vi "3D_Traverse_move.vi"(0 "Mode":T4=enum."Read traverse position", 1 "Position":sgl[](array[numeric])=[0.0, 0.0, 0.0] format="%#.2f", 2 "Extra command String":string, 3 "Work in Tunnel Coordinates":T2, 4 "Home":T1, 5 "Simulate/Run":T3=enum."Run VI", 6 "Route Checking?":bool=TRUE, 7 "Traverse name":string, 8 "Display Trav 2 Trav Error":bool=TRUE, 9 "Backlash Compensation?":bool=TRUE, 10 "Row Number":i32=-1, 11 "Last Part of Move?":bool=TRUE, 13 "Currently on Point":i32=-1) -> (12 "Model:    Roll        Pitch         Yaw  (deg)":sgl[](array[numeric]) caption="ModelRollPitchYaw (deg)" format="%#.2f", 14 "Trav Position achieved":sgl[](array[numeric]) format="%#.2f", 19 "Error String":string)   [LabVIEW 2016]
uses:
  Trav_mode.ctl
  Controls/User_Specific_mode.ctl
  Controls/Tunnel_Coordinates.ctl
  Controls/Home.ctl
  ADAM Client/Sub VIs/ADAM Controls/Quick_local_ADAM_Table.ctl
  Route mapping/Route_Display_Mode.ctl
  Controls/In_Range.ctl
  Globals/Trav_pos_global.vi
  Globals/Preference_global.vi
  Globals/Constants_global.vi
  Route mapping/Route_mapping_global.vi
panel:
  in  "Position Offset":sgl[](array[numeric])=[0.0, 0.0, 0.0] step=1 format="%#.2f"
  out "Traverses Available":string[](array[string])
  in  "Traverse":u16(ring) items=["EnFlo_Stack", "EnFlo_Trav1", "EnFlo_Trav3", "EnFlo_Trav4", "EnFlo_Tunnel", "EnFlo_Turntable"]
  # "X                Y                   Z"
  # "X                Y                   Z"
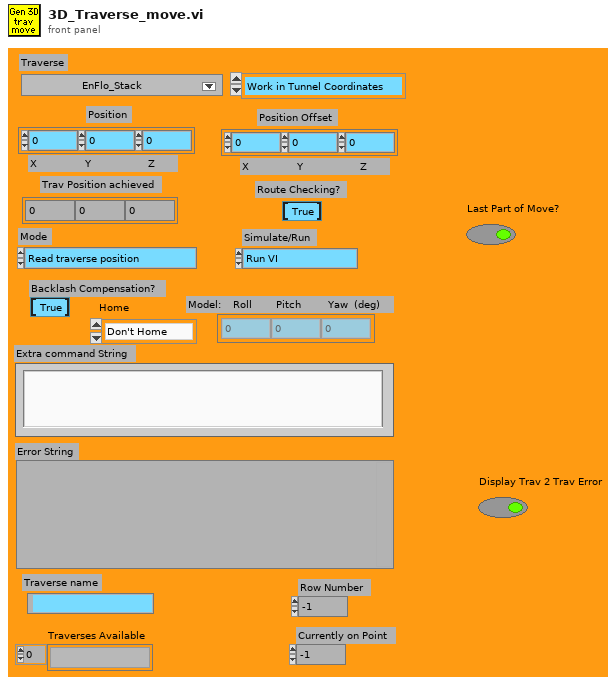
[diagram p1: front panel]
types:
  T1 = typedef "Home.ctl" = enum16{"Don't Home", "Home  +X", "Home  -X", "Home  +Y", "Home  -Y", "Home  +Z", "Home  -Z"}
  T2 = typedef "Tunnel_Coordinates.ctl" = enum16{"Work in Tunnel Coordinates", "Work in Model Coordinates"}
  T3 = typedef "User_Specific_mode.ctl" = enum16{"Check VI only", "Run VI"}
  T4 = typedef "Trav_mode.ctl" = enum16{"Move traverse", "Read traverse position", "Teach Position"}
  T5 = enum16{"To Traverse Coordinates", "To User Coordinates"}
  T6 = typedef "Quick_local_ADAM_Table.ctl" = enum16{"Read Global", "Load Global From ADAM Table", "Write Global"}
  T7 = typedef "Route_Display_Mode.ctl" = enum16{"Display View Always", "Display View on Crash"}
  T8 = typedef "In_Range.ctl" = enum16{"%", "±", "% & ±"}
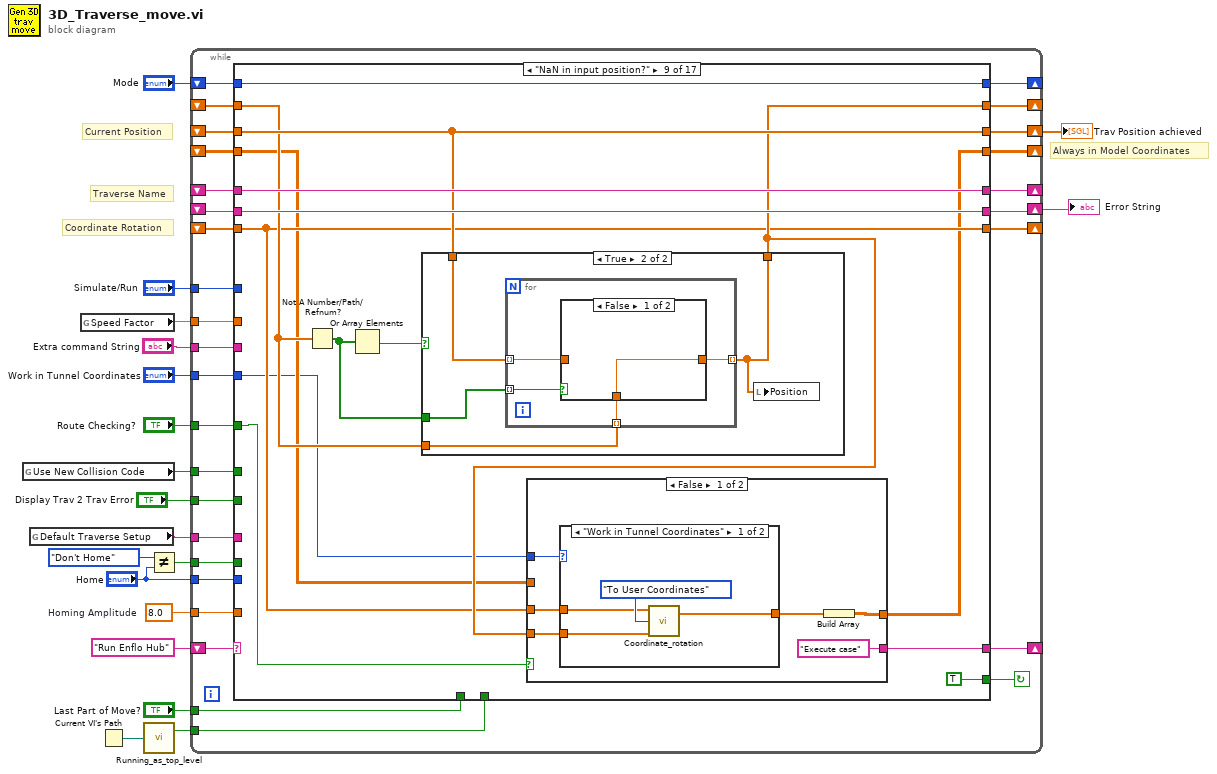
[diagram p0: block diagram]
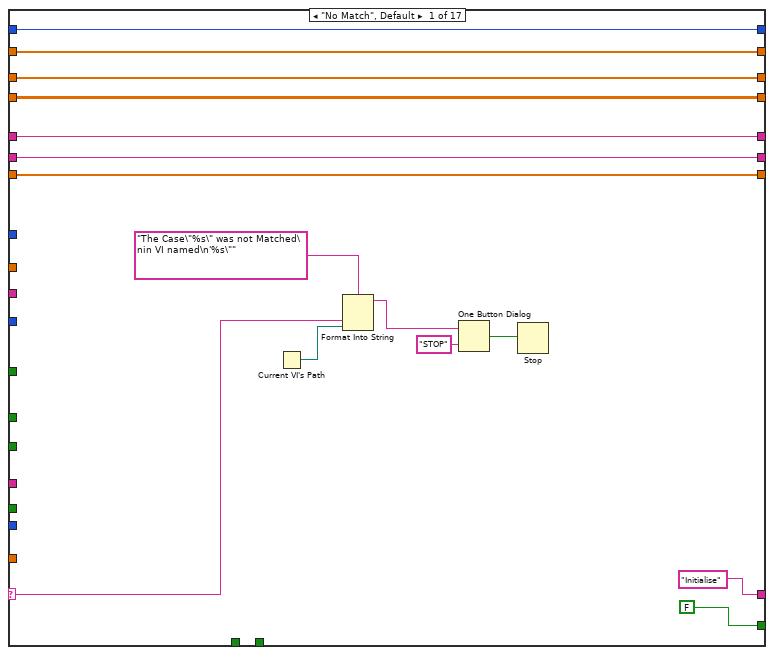
[diagram p2: hidden frame]
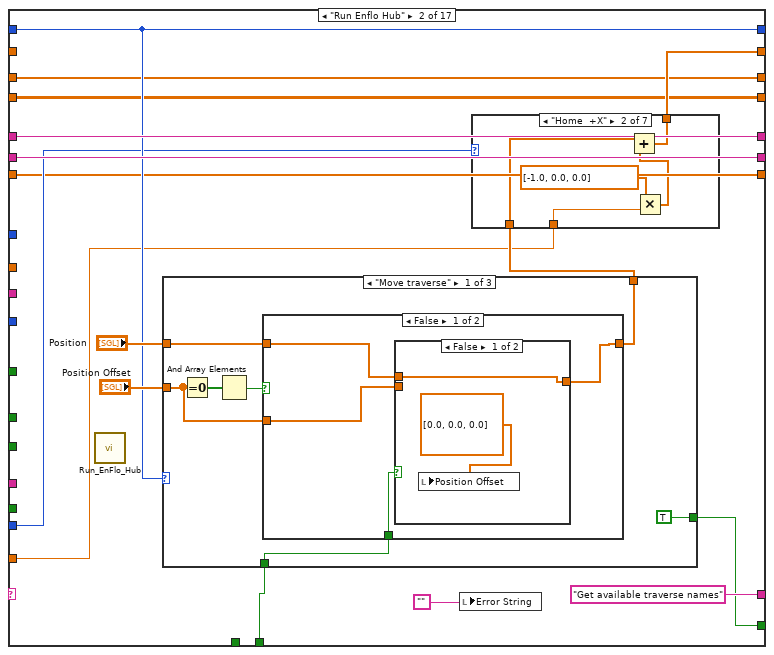
[diagram p3: hidden frame]
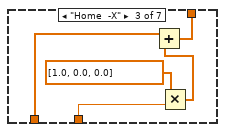
[diagram p5: hidden frame]
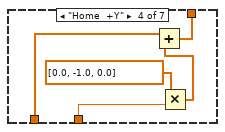
[diagram p6: hidden frame]
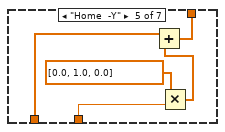
[diagram p7: hidden frame]
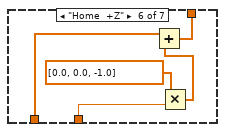
[diagram p8: hidden frame]
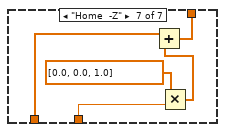
[diagram p9: hidden frame]
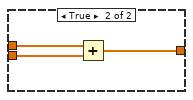
[diagram p10: hidden frame]
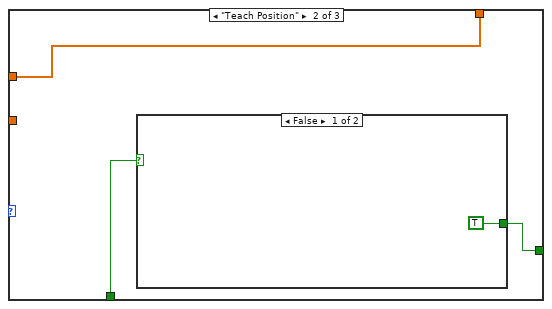
[diagram p12: hidden frame]
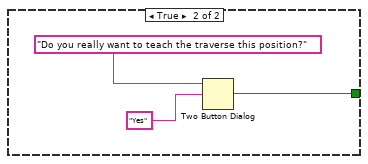
[diagram p13: hidden frame]
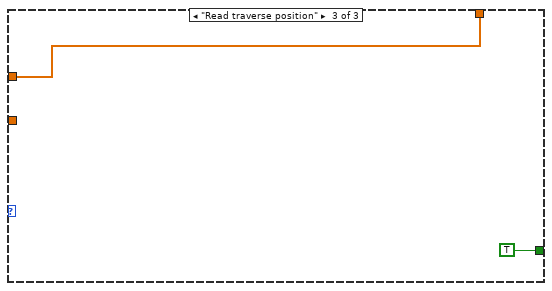
[diagram p14: hidden frame]
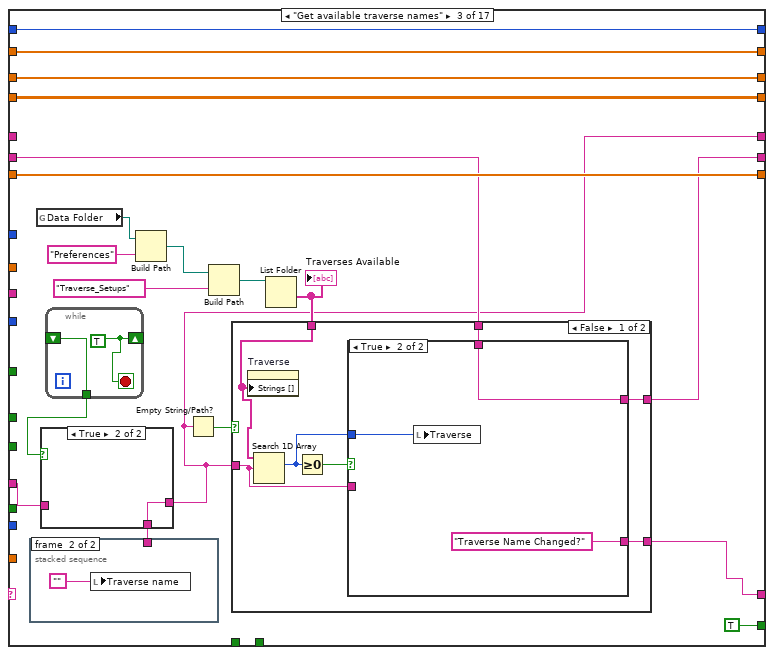
[diagram p15: hidden frame]
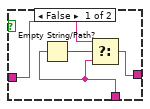
[diagram p16: hidden frame]
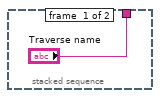
[diagram p17: hidden frame]
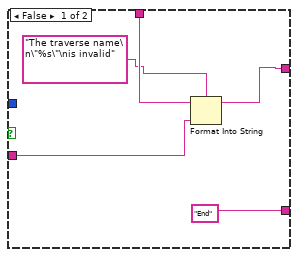
[diagram p18: hidden frame]
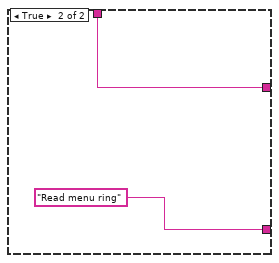
[diagram p19: hidden frame]
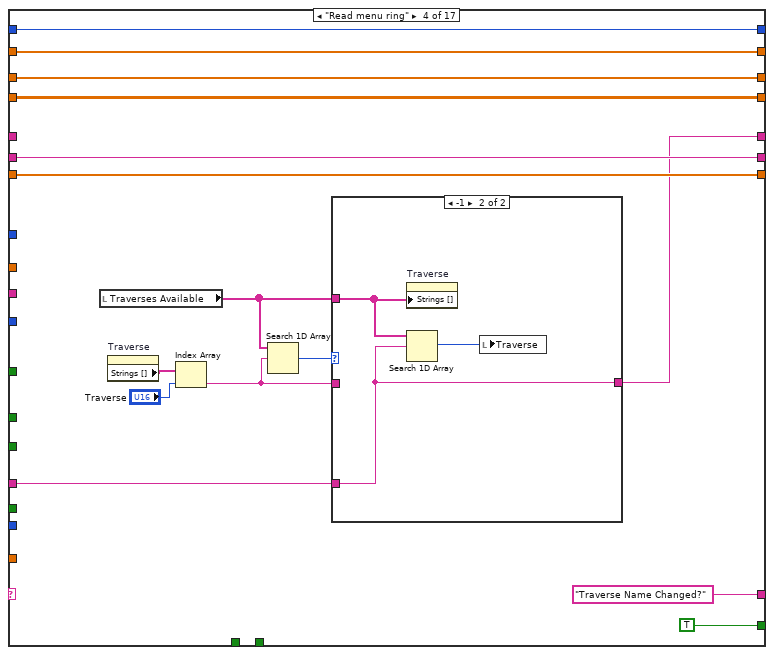
[diagram p20: hidden frame]
diagram:
  w10 = sgl 8.0  # Homing Amplitude
  # "Always in Model Coordinates"
  # "Current Position"
  # "Coordinate Rotation"
  # "Traverse Name"
  n1 = global read "Preference_global.vi" "Use New Collision Code"() -> (w6:bool)
  n2 = global read "Trav_pos_global.vi" "Default Traverse Setup"() -> (w12:string)
  n3 = global read "Trav_pos_global.vi" "Speed Factor"() -> (w16:sgl)
  n4 = Current VI's Path() -> (path=w4:path)
  n5 = call "Running_as_top_level.vi"("Vi path name"=w4) -> ("Top Level"=w3:bool)  [unwired: 1 out]
  n6 = Not Equal?(x=Home."Don't Home" ("Home"), y="Home") -> (x != y?=w7:bool)
  n7 = while {
    shift-left: "Run Enflo Hub" -> [w47]
    shift-right: [w48] -> _
    shift-right: [w45] -> _
    shift-left: _ -> [w43]
    tunnel: "Simulate/Run" -> [w46]
    shift-right: [w44] -> w17
    shift-left: _ -> [w42]
    shift-right: [w40] -> _
    shift-left: _ -> [w41]
    shift-right: [w37] -> _
    shift-left: _ -> [w36]
    shift-right: [w38] -> w13
    shift-left: _ -> [w39]
    tunnel: w16 -> [w35]
    tunnel: "Work in Tunnel Coordinates" -> [w34]
    tunnel: "Route Checking?" -> [w33]
    tunnel: w12 -> [w32]
    shift-right: [w31] -> _
    shift-left: _ -> [w30]
    shift-right: [w28] -> _
    shift-left: "Mode" -> [w29]
    tunnel: "Home" -> [w27]
    tunnel: w10 -> [w26]
    tunnel: w7 -> [w25]
    tunnel: w6 -> [w24]
    tunnel: "Last Part of Move?" -> [w23]
    tunnel: w3 -> [w22]
    tunnel: "Extra command String" -> [w21]
    tunnel: "Display Trav 2 Trav Error" -> [w20]
    stop <- w49 continue-if-true
    n8 = case shown="\"NaN in input position?\"" w47 {
      selector: w47 -> [w50 _ _ _ _ _ _ _ _ _ _ _ _ _ _ _ _]
      tunnel: [FALSE w76 TRUE TRUE TRUE TRUE w292 TRUE ("T button?") TRUE ("T button?") w395 TRUE w550 w577 TRUE TRUE TRUE FALSE] -> w49
      tunnel: ["Initialise" "Get available traverse names" w148 "Traverse Name Changed?" "Mode" w261 w299 "NaN in input position?" w353 w396 w449 "Display Traverse Views" w584 "Update Position Globals" "Tidy up" "End" "End"] -> w48
      tunnel: w46 -> [_ _ _ _ w226 w262 w304 _ _ w404 w445 _ w582 _ w681 w723 w821]
      tunnel: [w57 w79 w140 w184 w221 w254 w308 w340 w366 w406 w444 w555 w589 w631 w680 w728 w817] -> w45
      tunnel: [w56 w78 w146 w196 "" w263 w293 "" w363 w399 w453 w547 w586 w616 w684 w730 w824] -> w44
      tunnel: w43 -> [w57 w79 _ _ w221 w254 w308 w340 w366 w406 w444 w555 w589 w631 w680 w728 w817]
      tunnel: w42 -> [w56 w78 w145 w196 _ w263 _ _ w363 w401 _ w548 w586 _ w684 w731 w824]
      tunnel: w41 -> [w55 w67 w157 w195 _ w264 w307 w343 w356 w402 w436 w543 w592 w629 w677 w733 w818]
      tunnel: [w55 w67 w157 w195 w204 w264 w307 w343 w356 w402 w436 w543 w592 w629 w677 w733 w818] -> w40
      tunnel: w39 -> [w54 w66 w156 w194 w227 w256 w305 _ w362 w398 w451 w554 w591 _ w679 w732 w819]
      tunnel: [w54 w66 w156 w194 w227 w256 w297 w342 w362 w398 w452 w554 w591 w627 w679 w732 w819] -> w38
      tunnel: [w53 w65 w155 w193 w206 w265 w309 w346 w355 w407 w439 w553 w590 w621 w685 w734 w825] -> w37
      tunnel: w36 -> [w53 w65 w155 w193 _ w265 w309 w346 w354 w407 _ w553 w590 w621 w685 w734 w825]
      tunnel: w35 -> [_ _ _ _ _ _ _ _ _ _ _ _ _ w630 _ _ _]
      tunnel: w34 -> [_ _ _ _ w205 w258 w291 w344 w352 w403 w454 w544 _ w610 w678 _ w820]
      tunnel: w33 -> [_ _ _ _ _ _ _ _ w358 _ _ _ _ w625 _ _ _]
      tunnel: w32 -> [_ _ w139 w188 _ _ _ _ _ _ _ _ _ _ _ _ _]
      tunnel: [w52 w71 w143 w186 w203 w255 w298 w341 w357 w405 w443 w546 w576 w624 w683 w727 w822] -> w31
      tunnel: w30 -> [w52 _ w143 w186 w203 w255 w298 w341 w359 w405 w443 w546 w576 w624 w683 w727 w822]
      tunnel: w29 -> [w51 w73 w142 w185 w222 w253 w296 w336 w364 w408 w442 w545 w575 w623 w682 w726 w814]
      tunnel: [w51 w73 w142 w185 w223 w253 w296 w336 w364 w408 w442 w545 w575 w623 w682 w726 w814] -> w28
      tunnel: w27 -> [_ w70 _ _ _ _ _ _ _ _ w441 _ _ w617 _ w725 _]
      tunnel: w26 -> [_ w69 _ _ _ _ _ _ _ _ w438 _ _ _ _ w724 _]
      tunnel: w25 -> [_ _ _ _ _ _ _ _ _ _ _ _ _ _ _ w722 _]
      tunnel: w24 -> [_ _ _ _ w211 _ _ _ _ _ w437 _ _ _ _ _ w815]
      tunnel: w23 -> [_ _ _ _ _ _ _ _ _ _ _ _ _ w612 _ _ _]
      tunnel: w22 -> [_ w68 _ _ w208 _ _ _ _ _ _ w542 _ w615 _ _ _]
      tunnel: w21 -> [_ _ _ _ _ _ w295 _ _ _ _ _ _ w611 _ _ _]
      tunnel: w20 -> [_ _ _ _ _ _ _ _ _ w394 _ _ _ _ _ _ _]
      frame "No Match", Default {
        n9 = Current VI's Path() -> (path=w59:path)
        n10 = Format Into String(format string="The Case\"%s\" was not Matched\nin VI named\n'%s\"" ("Format String"), w50, w59) -> (resulting string=w62:string)  [unwired: 2 in, 1 out]
        n11 = One Button Dialog(message=w62, button name ("OK")="STOP") -> (true=w60:bool)
        n12 = Stop(stop? (T)=w60) -> ()
      }
      frame "Run Enflo Hub" {
        n13 = call "Run_EnFlo_Hub.vi"() -> ()  [unwired: 1 in, 7 out]
        n14 = case shown="\"Move traverse\"" w73 {
          tunnel: [TRUE ("T button?") w131 TRUE ("T button?")] -> w76
          tunnel: [w115 w130 w137] -> w72
          tunnel: "Position" -> [w114 w130 w137]
          tunnel: "Position Offset" -> [w113 _ _]
          tunnel: w68 -> [w112 w129 _]
          frame "Move traverse" {
            n15 = Equal To 0?(x=w113) -> (x = 0?=w117:bool[])
            n16 = And Array Elements(Boolean array=w117) -> (logical AND=w116:bool)
            n17 = case shown="False" w116 {
              tunnel: [w120 w128] -> w115
              tunnel: w114 -> [w122 w128]
              tunnel: w113 -> [w121 _]
              tunnel: w112 -> [w119 _]
              frame False {
                n18 = case shown="False" w119 {
                  tunnel: w122 -> [w124 w127]
                  tunnel: w121 -> [_ w126]
                  tunnel: [w124 w125] -> w120
                  frame False {
                    n19 = local write "Position Offset"(sgl[] [0.0, 0.0, 0.0] ("Position Increment")) -> ()
                  }
                  frame True {
                    n20 = Add(x=w127, y=w126) -> (x+y=w125:sgl[])
                  }
                }
              }
              frame True {
              }
            }
          }
          frame "Teach Position" {
            n21 = case shown="False" w129 {
              tunnel: [TRUE ("T button?") w133] -> w131
              frame False {
              }
              frame True {
                n22 = Two Button Dialog(message="Do you really want to teach the traverse this position?", 2:"Yes" ("T button name (\"OK\")")) -> (T button?=w133:bool)  [unwired: 1 out]
              }
            }
          }
          frame "Read traverse position" {
          }
        }
        n23 = local write "Error String"("") -> ()
        n24 = case shown="\"Home  +X\"" w70 {
          tunnel: [w81 w85 w90 w95 w100 w105 w110] -> w71
          tunnel: w72 -> [w81 w86 w91 w96 w101 w106 w111]
          tunnel: w69 -> [_ w82 w87 w92 w97 w102 w107]
          frame "Don't Home" {
          }
          frame "Home  +X" {
            n25 = Multiply(x=sgl[] [-1.0, 0.0, 0.0] ("y"), y=w82) -> (x*y=w83:sgl[])
            n26 = Add(x=w86, y=w83) -> (x+y=w85:sgl[])
          }
          frame "Home  -X" {
            n27 = Multiply(x=sgl[] [1.0, 0.0, 0.0] ("y"), y=w87) -> (x*y=w88:sgl[])
            n28 = Add(x=w91, y=w88) -> (x+y=w90:sgl[])
          }
          frame "Home  +Y" {
            n29 = Multiply(x=sgl[] [0.0, -1.0, 0.0] ("y"), y=w92) -> (x*y=w93:sgl[])
            n30 = Add(x=w96, y=w93) -> (x+y=w95:sgl[])
          }
          frame "Home  -Y" {
            n31 = Multiply(x=sgl[] [0.0, 1.0, 0.0] ("y"), y=w97) -> (x*y=w98:sgl[])
            n32 = Add(x=w101, y=w98) -> (x+y=w100:sgl[])
          }
          frame "Home  +Z" {
            n33 = Multiply(x=sgl[] [0.0, 0.0, -1.0] ("y"), y=w102) -> (x*y=w103:sgl[])
            n34 = Add(x=w106, y=w103) -> (x+y=w105:sgl[])
          }
          frame "Home  -Z" {
            n35 = Multiply(x=sgl[] [0.0, 0.0, 1.0] ("y"), y=w107) -> (x*y=w108:sgl[])
            n36 = Add(x=w111, y=w108) -> (x+y=w110:sgl[])
          }
        }
      }
      frame "Get available traverse names" {
        n37 = stacked-sequence {
          tunnel: ["Traverse name" _] -> w138
          frame #0 {
          }
          frame #1 {
            n38 = local write "Traverse name"("") -> ()
          }
        }
        n39 = global read "Constants_global.vi" "Data Folder"() -> (w151:path)
        n40 = while {
          shift-right: [w165] -> _
          shift-left: _ -> [w166]
          tunnel: [w166] -> w141
          stop <- w165 stop-if-true
          w165 = TRUE
        }
        n41 = case shown="True" w141 {
          tunnel: [w160 w162] -> w140
          tunnel: w139 -> [w159 _]
          tunnel: w138 -> [w158 w162]
          frame False {
            n42 = Empty String/Path?(string/path=w158) -> (empty?=w161:bool)
            n43 = Select(t=w159, s=w161, f=w158) -> (s? t:f=w160:string)
          }
          frame True {
          }
        }
        n44 = Build Path(base path=w151, name or relative path="Preferences") -> (appended path=w153:path)
        n45 = Empty String/Path?(string/path=w140) -> (empty?=w149:bool)
        n46 = Build Path(base path=w153, name or relative path="Traverse_Setups") -> (appended path=w154:path)
        n47 = List Folder(path=w154) -> (folder names=w147:string[])  [unwired: 1 in, 5 out]
        "Traverses Available" <- w147
        n48 = case shown="False" w149 {
          tunnel: [w170 "Read menu ring"] -> w148
          tunnel: w147 -> [w167 _]
          tunnel: w140 -> [w173 _]
          tunnel: [w172 w182] -> w146
          tunnel: w145 -> [w171 w182]
          frame False {
            n49 = property on="Traverse" class="Ring (strict)"("Strings []"=w167) -> ()  [unwired: 2 in, 2 out]
            n50 = Search 1D Array(1D array=w167, element=w173) -> (index of element=w168:i32)  [unwired: 1 out]
            n51 = Greater Or Equal To 0?(x=w168) -> (x >= 0?=w169:bool)
            n52 = case shown="True" w169 {
              tunnel: w173 -> [w178 _]
              tunnel: [w175 w181] -> w172
              tunnel: w171 -> [w177 w181]
              tunnel: ["End" "Traverse Name Changed?"] -> w170
              tunnel: w168 -> [_ w179]
              frame False {
                n53 = Format Into String(format string="The traverse name\n\"%s\"\nis invalid", initial string=w177, w178) -> (resulting string=w175:string)  [unwired: 1 in, 1 out]
              }
              frame True {
                n54 = local write "Traverse"(w179) -> ()
              }
            }
          }
          frame True {
          }
        }
      }
      frame "Read menu ring" {
        n55 = local read "Traverses Available"() -> (w189:string[])
        n56 = property on="Traverse" class="Ring (strict)"() -> ("Strings []"=w192:string[])  [unwired: 2 in, 2 out]
        n57 = Index Array(array=w192, index="Traverse") -> (element=w187:string)
        n58 = Search 1D Array(1D array=w189, element=w187) -> (index of element=w190:i32)  [unwired: 1 out]
        n59 = case shown="-1" w190 {
          tunnel: w189 -> [_ w202]
          tunnel: w188 -> [_ w200]
          tunnel: [w199 w200] -> w184
          tunnel: w187 -> [w199 _]
          frame 0, Default {
          }
          frame -1 {
            n60 = property on="Traverse" class="Ring (strict)"("Strings []"=w202) -> ()  [unwired: 2 in, 2 out]
            n61 = Search 1D Array(1D array=w202, element=w200) -> (index of element=w201:i32)  [unwired: 1 out]
            n62 = local write "Traverse"(w201) -> ()
          }
        }
      }
      frame "Traverse Name Changed?" {
        n63 = call "Rig_Pict_Display_Pref.vi"("Traverse Name"=w221) -> ("Roll Pitch Yaw ADAM Channels"=w220:string[])  [unwired: 3 in, 4 out]
        n64 = Build Array (concatenate)(w220, "EnFlo_Tunnel:Trav Origin:X Offset") -> (w218:string[])
        n65 = case shown="\"Run VI\"" w226 {
          tunnel: [w249 w251] -> w210
          tunnel: w218 -> [w250 w252]
          frame "Check VI only" {
            n66 = call "Read_Write_Local_table_Quick.vi"("Mode"=Quick_local_ADAM_Table."Read Global", "Ch names In"=w250) -> ("Numeric Values Out"=w249:dbl[])  [unwired: 1 in, 2 out]
          }
          frame "Run VI" {
            n67 = call "Get_Current_Scan_client.vi"("ADAM Ch Names"=w252) -> ("Numerical Values"=w251:dbl[])  [unwired: 3 out]
          }
        }
        n68 = To Single Precision Float(number=w210) -> (single precision float=w209:sgl[])
        n69 = Split 1D Array(array=w209, index=3) -> (first subarray=w216:sgl[], second subarray=w214:sgl[])
        n70 = global read "Route_mapping_global.vi" "Traverse Setup"() -> (w212:string)
        n71 = for {
          tunnel: w216 -> [w246] mode=indexing
          tunnel: [w244] -> w204 mode=indexing
          n72 = Not A Number/Path/Refnum?(number/path/refnum=w246) -> (NaN/Path/Refnum?=w247:bool)
          n73 = Select(t=sgl 0.0, s=w247, f=w246) -> (s? t:f=w244:sgl)
        }
        "Model:    Roll        Pitch         Yaw  (deg)" <- w204
        n74 = case shown="\"Work in Tunnel Coordinates\"" w205 {
          tunnel: [w233 w235] -> w207
          tunnel: w204 -> [w232 _]
          tunnel: w203 -> [w231 w235]
          frame "Work in Tunnel Coordinates" {
            n75 = call "Coordinate_rotation.vi"("Roll-Pitch-Yaw"=w232, "Input Position"=w231, "Mode"=T5."To User Coordinates") -> ("Output Position"=w233:sgl[])  [unwired: 2 in, 1 out]
          }
          frame "Work in Model Coordinates" {
          }
        }
        n76 = Build Array(w207) -> (w206:sgl[][])
        n77 = Index Array(array=w214) -> (element=w215:sgl)  [unwired: 1 in]
        n78 = global write "Trav_pos_global.vi" "Traverse Origin X Offset (mm)"(w215) -> ()
        n79 = Equal?(x=w212, y=w221) -> (x = y?=w213:bool)
        n80 = case shown="False" w213 {
          tunnel: w221 -> [w238 _]
          tunnel: [w236 FALSE ("Top Level")] -> w225
          tunnel: w211 -> [w237 _]
          tunnel: w208 -> [w236 _]
          frame False {
            n81 = case shown="True" w237 {
              tunnel: w238 -> [w239 w241]
              frame False {
                w240 = FALSE  # Show Panel?
                n82 = call "Traverse_Space.vi"("Show Panel?"=w240, "Traverse Setup"=w239) -> ()  [unwired: 1 in, 8 out]
              }
              frame True {
                w242 = FALSE  # Show Panel?
                n83 = call "Traverse_Space_for new collision code.vi"("Show Panel?"=w242, "Traverse Setup"=w241) -> ()  [unwired: 8 in, 1 out]
              }
            }
          }
          frame True {
          }
        }
        n84 = Select(t=Trav_mode."Read traverse position" ("Mode"), s=w225, f=w222) -> (s? t:f=w223:T4)
      }
      frame "Mode" {
        n85 = while {
          shift-right: [w269] -> _
          shift-left: _ -> [w268]
          tunnel: w258 -> [w269]
          tunnel: [w267] -> w257
          stop <- TRUE stop-if-true
          n86 = Equal?(x=w268, y=w269) -> (x = y?=w267:bool)
        }
        n87 = case shown="\"Run VI\"" w262 {
          tunnel: w253 -> [_ w276]
          tunnel: [w271 w275] -> w261
          tunnel: "Execute case" -> [_ w274]
          tunnel: "Read Current Position" -> [w271 w273]
          tunnel: w257 -> [_ _]
          tunnel: w254 -> [_ w272]
          frame "Check VI only" {
          }
          frame "Run VI" {
            n88 = case shown="\"Read traverse position\", Default" w276 {
              tunnel: [w288 w290] -> w275
              tunnel: w274 -> [_ w290]
              tunnel: w273 -> [w287 _]
              tunnel: w272 -> [w289 _]
              frame "Move traverse" {
                n89 = global read "Constants_global.vi" "Traverse folder"() -> (w284:path)
                n90 = Build Path(base path=w284, name or relative path=w289) -> (appended path=w286:path)
                n91 = Build Path(base path=w286, name or relative path="Motor_Pos.xls" ("Substring")) -> (appended path=w283:path)
                n92 = File/Directory Info(path=w283) -> (last mod=w281:timestamp)  [unwired: 1 in, 6 out]
                n93 = Get Date/Time In Seconds() -> (seconds since 1Jan1904=w282:timestamp)
                n94 = Subtract(x=w282, y=w281) -> (x-y=w280:dbl)
                n95 = Greater?(x=w280, y=40.0) -> (0:w278:bool)
                n96 = Select(t=w287, s=w278, f="Quick Read from file") -> (s? t:f=w288:string)
              }
              frame "Read traverse position", Default {
              }
            }
          }
        }
      }
      frame "Read Current Position" {
        n97 = case shown="\"Run VI\"" w304 {
          tunnel: w308 -> [w315 w329]
          tunnel: ["" w320] -> w293
          tunnel: w307 -> [_ w325]
          tunnel: [w316 w330] -> w306
          tunnel: w305 -> [_ w324]
          tunnel: w295 -> [_ w321]
          tunnel: w291 -> [_ w319]
          frame "Check VI only" {
            n98 = call "Read-Write_Check_Pos.vi"("Mode"=enum16{"Read", "Write"}."Read", "Traverse Name"=w315) -> ("Position Output"=w316:sgl[])  [unwired: 1 in]
          }
          frame "Run VI" {
            w323 = TRUE  # Last Part of Move?
            w328 = FALSE  # Route Checking?
            w327 = FALSE  # Backlash Compensation?
            n99 = call "TraverseControl_High.vi"("Mode"=Trav_mode."Read traverse position", "Route Checking?"=w328, "Home"=Home."Don't Home", "Traverse Name"=w329, "Extra command String"=w321, "Work in Tunnel Coordinates"=w319, "Model       Roll      Pitch       Yaw (deg)"=w325, "Position input XYZ"=w324, "Last Part of Move?"=w323, "Backlash Compensation?"=w327) -> ("Position Output XYZ"=w330:sgl[], "Error String"=w320:string)  [unwired: 4 in]
          }
        }
        n100 = Equal?(x=Trav_mode."Read traverse position" ("Mode"), y=w296) -> (x = y?=w302:bool)
        n101 = case shown="\"Work in Model Coordinates\"" w291 {
          tunnel: w306 -> [w331 w333]
          tunnel: [w331 w334] -> w297
          tunnel: w307 -> [_ w332]
          frame "Work in Tunnel Coordinates" {
          }
          frame "Work in Model Coordinates" {
            n102 = call "Coordinate_rotation.vi"("Roll-Pitch-Yaw"=w332, "Input Position"=w333, "Mode"=T5."To User Coordinates") -> ("Output Position"=w334:sgl[])  [unwired: 2 in, 1 out]
          }
        }
        n103 = Empty String/Path?(string/path=w293) -> (empty?=w294:bool)
        n104 = case shown="True" w294 {
          tunnel: w293 -> [w312 _]
          tunnel: [w310 TRUE] -> w292
          frame False {
            n105 = Match Pattern(string=w312, regular expression="Trav Axis Correction Error" ("string")) -> (offset past match=w311:i32)  [unwired: 4 out]
            n106 = Greater Or Equal To 0?(x=w311) -> (x >= 0?=w310:bool)
          }
          frame True {
          }
        }
        n107 = Select(t="Update Position Globals", s=w302, f="NaN in input position?") -> (s? t:f=w299:string)
      }
      frame "Quick Read from file" {
        n108 = call "Read_Traverse_Pos_File.vi"("Traverse Name"=w340) -> ("Tunnel Coordinates"=w339:sgl[])
        n109 = case shown="\"Work in Model Coordinates\"" w344 {
          tunnel: w339 -> [w347 w350]
          tunnel: [w347 w349] -> w342
          tunnel: w343 -> [_ w348]
          frame "Work in Tunnel Coordinates" {
          }
          frame "Work in Model Coordinates" {
            n110 = call "Coordinate_rotation.vi"("Roll-Pitch-Yaw"=w348, "Input Position"=w350, "Mode"=T5."To User Coordinates") -> ("Output Position"=w349:sgl[])  [unwired: 2 in, 1 out]
          }
        }
      }
      frame "NaN in input position?" {
        n111 = Not A Number/Path/Refnum?(number/path/refnum=w359) -> (NaN/Path/Refnum?=w361:bool[])
        n112 = Or Array Elements(Boolean array=w361) -> (logical OR=w360:bool)
        n113 = case shown="True" w360 {
          tunnel: w361 -> [_ w384]
          tunnel: w362 -> [_ w383]
          tunnel: w359 -> [w380 w382]
          tunnel: [w380 w381] -> w357
          frame False {
          }
          frame True {
            n114 = for {
              tunnel: w384 -> [w388] mode=indexing
              tunnel: w383 -> [w387] mode=indexing
              tunnel: [w386] -> w381 mode=indexing
              tunnel: w382 -> [w385] mode=indexing
              n115 = case shown="False" w388 {
                tunnel: w387 -> [_ w390]
                tunnel: [w389 w390] -> w386
                tunnel: w385 -> [w389 _]
                frame False {
                }
                frame True {
                }
              }
            }
            n116 = local write "Position"(w381) -> ()
          }
        }
        n117 = case shown="False" w358 {
          tunnel: w357 -> [w372 _]
          tunnel: w356 -> [w371 _]
          tunnel: [w369 w379] -> w355
          tunnel: w354 -> [_ w379]
          tunnel: ["Execute case" "Perform Route Check"] -> w353
          tunnel: w352 -> [w367 _]
          frame False {
            n118 = case shown="\"Work in Tunnel Coordinates\"" w367 {
              tunnel: w372 -> [w375 w377]
              tunnel: w371 -> [w374 _]
              tunnel: [w373 w377] -> w370
              frame "Work in Tunnel Coordinates" {
                n119 = call "Coordinate_rotation.vi"("Roll-Pitch-Yaw"=w374, "Input Position"=w375, "Mode"=T5."To User Coordinates") -> ("Output Position"=w373:sgl[])  [unwired: 2 in, 1 out]
              }
              frame "Work in Model Coordinates" {
              }
            }
            n120 = Build Array(w370) -> (w369:sgl[][])
          }
          frame True {
          }
        }
      }
      frame "Perform Route Check" {
        n121 = Select(t=2, s=w394, f=1) -> (s? t:f=w391:i32)
        n122 = for {
          N: w391 -> [_]
          tunnel: w406 -> [w421]
          tunnel: w405 -> [w420]
          tunnel: w404 -> [w419]
          tunnel: w403 -> [w418]
          tunnel: w402 -> [w417]
          tunnel: [w414] -> w400
          tunnel: w398 -> [w416]
          tunnel: [w413] -> w397
          i -> [w415]
          stop <- w413 stop-if-true
          n123 = case shown="0, Default" w415 {
            tunnel: w421 -> [w428 w435]
            tunnel: w420 -> [w427 w434]
            tunnel: w419 -> [w426 w433]
            tunnel: w418 -> [w425 w432]
            tunnel: w417 -> [w424 w431]
            tunnel: [w423 w430] -> w414
            tunnel: w416 -> [w422 w429]
            frame 1 {
              n124 = call "Traverse_to_Traverse_Collision.vi"("Current Position"=w422, "Traverse Name"=w428, "Model  Roll        Pitch       Yaw (deg)"=w424, "Work in Tunnel Coordinates"=w425, "Simulate/Run"=w426, "New Position"=w427) -> ("Error String"=w423:string)  [unwired: 5 in]
            }
            frame 0, Default {
              n125 = call "Traverse_to_Traverse_Collision.vi"("Current Position"=w429, "Traverse Name"=w435, "Model  Roll        Pitch       Yaw (deg)"=w431, "Work in Tunnel Coordinates"=w432, "Simulate/Run"=w433, "New Position"=w434) -> ("Error String"=w430:string)  [unwired: 5 in]
            }
          }
          n126 = Empty String/Path?(string/path=w414) -> (empty?=w413:bool)
        }
        n127 = case shown="False" w397 {
          tunnel: ["Route Error" "Perform Route Check_2" ("f")] -> w396
          tunnel: [w409 TRUE] -> w395
          tunnel: w394 -> [w409 _]
          frame False {
          }
          frame True {
          }
        }
        n128 = Concatenate Strings(w401, w400) -> (w399:string)
      }
      frame "Perform Route Check_2" {
        n129 = case shown="True" w437 {
          tunnel: w454 -> [w464 w482]
          tunnel: [w455 w480] -> w453
          tunnel: w451 -> [w463 w479]
          tunnel: w445 -> [w458 w478]
          tunnel: w444 -> [w459 w477]
          tunnel: w443 -> [w462 w476]
          tunnel: [w456 w474] -> w440
          tunnel: w436 -> [w457 w473]
          frame True {
            n130 = case shown="\"Work in Model Coordinates\"" w464 {
              tunnel: w457 -> [_ w471]
              tunnel: w462 -> [w465 w467]
              tunnel: w463 -> [w466 w470]
              tunnel: [w465 w469] -> w460
              tunnel: [w466 w468] -> w461
              frame "Work in Tunnel Coordinates" {
              }
              frame "Work in Model Coordinates" {
                w472 = T5."To Traverse Coordinates" ("Mode")
                n131 = call "Coordinate_rotation.vi"("Roll-Pitch-Yaw"=w471, "Input Position"=w470, "Mode"=w472) -> ("Output Position"=w468:sgl[])  [unwired: 2 in, 1 out]
                n132 = call "Coordinate_rotation.vi"("Roll-Pitch-Yaw"=w471, "Input Position"=w467, "Mode"=w472) -> ("Output Position"=w469:sgl[])  [unwired: 2 in, 1 out]
              }
            }
            n133 = call "Check_with_Jump_PN.vi"("Current position"=w461, "Traverse Name"=w459, "Simulate/Run"=w458, "New Position"=w460, "Model       Roll      Pitch       Yaw (deg)"=w457) -> ("Error Comments"=w455:string, "Steps"=w456:sgl[][])  [unwired: 9 in]
          }
          frame False {
            n134 = case shown="\"Work in Tunnel Coordinates\"" w482 {
              tunnel: w473 -> [w487 _]
              tunnel: w476 -> [w483 w489]
              tunnel: w479 -> [w486 w490]
              tunnel: [w485 w489] -> w475
              tunnel: [w484 w490] -> w481
              frame "Work in Tunnel Coordinates" {
                w488 = T5."To User Coordinates" ("Mode")
                n135 = call "Coordinate_rotation.vi"("Roll-Pitch-Yaw"=w487, "Input Position"=w486, "Mode"=w488) -> ("Output Position"=w484:sgl[])  [unwired: 2 in, 1 out]
                n136 = call "Coordinate_rotation.vi"("Roll-Pitch-Yaw"=w487, "Input Position"=w483, "Mode"=w488) -> ("Output Position"=w485:sgl[])  [unwired: 2 in, 1 out]
              }
              frame "Work in Model Coordinates" {
              }
            }
            n137 = call "Check_with_Jump.vi"("Current position"=w481, "Traverse Name"=w477, "Simulate/Run"=w478, "New Position"=w475, "Model       Roll      Pitch       Yaw (deg)"=w473) -> ("Error Comments"=w480:string, "Steps"=w474:sgl[][])  [unwired: 9 in]
          }
        }
        n138 = case shown="\"Home  +Y\"" w441 {
          tunnel: w440 -> [w491 w498 w506 w514 w522 w530 w538]
          tunnel: [w491 w497 w505 w513 w521 w529 w537] -> w439
          tunnel: w438 -> [_ w492 w500 w508 w516 w524 w532]
          frame "Don't Home" {
          }
          frame "Home  +X" {
            n139 = for {
              tunnel: [w499] -> w496
              tunnel: w498 -> [w499] mode=indexing
            }
            n140 = Multiply(x=dbl[] [2.0, 0.0, 0.0] ("y"), y=w492) -> (x*y=w493:dbl[])
            n141 = Add(x=w496, y=w493) -> (x+y=w495:dbl[])
            n142 = Build Array (concatenate)(w498, w495) -> (w497:dbl[][])
          }
          frame "Home  -X" {
            n143 = for {
              tunnel: [w507] -> w504
              tunnel: w506 -> [w507] mode=indexing
            }
            n144 = Multiply(x=dbl[] [-2.0, 0.0, 0.0] ("y"), y=w500) -> (x*y=w501:dbl[])
            n145 = Add(x=w504, y=w501) -> (x+y=w503:dbl[])
            n146 = Build Array (concatenate)(w506, w503) -> (w505:dbl[][])
          }
          frame "Home  +Y" {
            n147 = for {
              tunnel: [w515] -> w512
              tunnel: w514 -> [w515] mode=indexing
            }
            n148 = Multiply(x=dbl[] [0.0, 2.0, 0.0] ("y"), y=w508) -> (x*y=w509:dbl[])
            n149 = Add(x=w512, y=w509) -> (x+y=w511:dbl[])
            n150 = Build Array (concatenate)(w514, w511) -> (w513:dbl[][])
          }
          frame "Home  -Y" {
            n151 = for {
              tunnel: [w523] -> w520
              tunnel: w522 -> [w523] mode=indexing
            }
            n152 = Multiply(x=dbl[] [0.0, -2.0, 0.0] ("y"), y=w516) -> (x*y=w517:dbl[])
            n153 = Add(x=w520, y=w517) -> (x+y=w519:dbl[])
            n154 = Build Array (concatenate)(w522, w519) -> (w521:dbl[][])
          }
          frame "Home  +Z" {
            n155 = for {
              tunnel: [w531] -> w528
              tunnel: w530 -> [w531] mode=indexing
            }
            n156 = Multiply(x=dbl[] [0.0, 0.0, 2.0] ("y"), y=w524) -> (x*y=w525:dbl[])
            n157 = Add(x=w528, y=w525) -> (x+y=w527:dbl[])
            n158 = Build Array (concatenate)(w530, w527) -> (w529:dbl[][])
          }
          frame "Home  -Z" {
            n159 = for {
              tunnel: [w539] -> w536
              tunnel: w538 -> [w539] mode=indexing
            }
            n160 = Multiply(x=dbl[] [0.0, 0.0, -2.0] ("y"), y=w532) -> (x*y=w533:dbl[])
            n161 = Add(x=w536, y=w533) -> (x+y=w535:dbl[])
            n162 = Build Array (concatenate)(w538, w535) -> (w537:dbl[][])
          }
        }
        n163 = Empty String/Path?(string/path=w453) -> (empty?=w446:bool)
        n164 = case shown="True" w446 {
          tunnel: [w540 w541] -> w452
          tunnel: w451 -> [w540 _]
          tunnel: w443 -> [_ w541]
          frame False {
          }
          frame True {
          }
        }
        n165 = Select(t="Display Traverse Views", s=w446, f="Route Error") -> (s? t:f=w449:string)
      }
      frame "Route Error" {
        n166 = global read "Trav_pos_global.vi" "Jump Bad Positions?"() -> (w552:bool)
        n167 = case shown="True" w552 {
          tunnel: w546 -> [_ w561]
          tunnel: [TRUE w560] -> w550
          tunnel: w544 -> [_ w559]
          tunnel: w543 -> [_ w558]
          tunnel: w542 -> [_ w557]
          frame False {
          }
          frame True {
            n168 = case shown="False" w557 {
              tunnel: w561 -> [w563 _]
              tunnel: [FALSE TRUE] -> w560
              tunnel: w559 -> [w565 _]
              tunnel: w558 -> [w562 _]
              frame False {
                n169 = case shown="\"Work in Tunnel Coordinates\"" w565 {
                  tunnel: [w570 w573] -> w564
                  tunnel: w563 -> [w571 w573]
                  tunnel: w562 -> [w569 _]
                  frame "Work in Tunnel Coordinates" {
                    n170 = call "Coordinate_rotation.vi"("Roll-Pitch-Yaw"=w569, "Input Position"=w571, "Mode"=T5."To User Coordinates") -> ("Output Position"=w570:sgl[])  [unwired: 2 in, 1 out]
                  }
                  frame "Work in Model Coordinates" {
                  }
                }
                n171 = global read "Trav_pos_global.vi" "Jumped Positions"() -> (w567:dbl[][])
                n172 = Build Array (concatenate)(w564, w567) -> (w566:dbl[][])
                n173 = global write "Trav_pos_global.vi" "Jumped Positions"(w566) -> ()
              }
              frame True {
              }
            }
          }
        }
        n174 = Concatenate Strings("Route Checking Error\n" ("string"), w548) -> (w547:string)
      }
      frame "Display Traverse Views" {
        n175 = global read "Route_mapping_global.vi" "Display Mode"() -> (w588:T7)
        n176 = Equal?(x=w582, y=User_Specific_mode."Check VI only" ("Simulate/Run")) -> (x = y?=w581:bool)
        n177 = Empty String/Path?(string/path=w586) -> (empty?=w577:bool)
        n178 = Equal?(x=w588, y=Route_Display_Mode."Display View Always" ("Display Mode")) -> (x = y?=w585:bool)
        n179 = Not(x=w577) -> (.not. x?=w578:bool)
        n180 = Or(x=w585, y=w578) -> (x .or. y?=w580:bool)
        n181 = And(x=w581, y=w580) -> (x .and. y?=w579:bool)
        n182 = case shown="True" w579 {
          tunnel: w590 -> [_ w601]
          tunnel: w589 -> [_ w600]
          tunnel: w586 -> [_ w597]
          tunnel: w577 -> [_ w595]
          frame False {
          }
          frame True {
            n183 = Not(x=w595) -> (.not. x?=w596:bool)
            n184 = for {
              tunnel: w601 -> [w608] mode=indexing
              tunnel: w600 -> [w607]
              tunnel: "Currently on Point" -> [w606]
              tunnel: "Row Number" -> [w605]
              tunnel: w597 -> [w604]
              tunnel: w596 -> [w602]
              n185 = Build Array(w608) -> (w609:dbl[][])
              n186 = call "Display_Trav_Views.vi"("Current Probe Position"=w609, "Traverse Name"=w607, "Currently on point"=w606, "Open Front Panel"=TRUE, "Error Comments"=w604, "Crash?"=w602, "Row Number"=w605) -> ()  [unwired: 4 out]
            }
          }
        }
        n187 = case shown="\"Run VI\"" w582 {
          tunnel: ["Update Position Globals" "Execute case"] -> w584
          frame "Check VI only" {
          }
          frame "Run VI" {
          }
        }
      }
      frame "Execute case" {
        n188 = Array Size(array=w621) -> (size(s)=w622:i32[])
        n189 = Index Array(array=w622) -> (element=w620:i32)  [unwired: 1 in]
        n190 = Decrement(x=w620) -> (x-1=w619:i32)
        n191 = Select(t=TRUE, s=w615, f=w612) -> (s? t:f=w613:bool)
        n192 = for {
          tunnel: w631 -> [w651]
          tunnel: w621 -> [w657] mode=indexing
          tunnel: w630 -> [w650]
          tunnel: w623 -> [w653]
          tunnel: w629 -> [w648]
          tunnel: [w655] -> w628
          tunnel: [w649] -> w616
          tunnel: w625 -> [w652]
          tunnel: w619 -> [w644]
          tunnel: w617 -> [w638]
          tunnel: "Backlash Compensation?" -> [w642]
          tunnel: w613 -> [w637]
          tunnel: w611 -> [w636]
          tunnel: w610 -> [w633]
          i -> [w643]
          stop <- w647 continue-if-true
          w639 = Home."Don't Home" ("Home")
          n193 = Not Equal?(x=w638, y=w639) -> (x != y?=w640:bool)
          n194 = Subtract(x=w644, y=w643) -> (x-y=w635:i32)
          n195 = case shown="0" w635 {
            tunnel: [w661 w665 w669] -> w646
            tunnel: [w659 w664 w666] -> w645
            tunnel: w642 -> [w663 _ w671]
            tunnel: [w658 w665 FALSE ("f")] -> w641
            tunnel: w640 -> [w660 _ w667]
            tunnel: w639 -> [_ w664 w666]
            tunnel: w638 -> [w659 _ _]
            tunnel: w637 -> [w658 _ _]
            frame 0 {
              n196 = Select(t=FALSE, s=w660, f=w663) -> (s? t:f=w661:bool)
            }
            frame Default {
              w665 = FALSE ("f")
            }
            frame 1 {
              n197 = Select(t=w671, s=w667, f=FALSE) -> (s? t:f=w669:bool)
            }
          }
          n198 = call "Coordinate_rotation.vi"("Roll-Pitch-Yaw"=w648, "Input Position"=w657, "Mode"=T5."To Traverse Coordinates") -> ("Output Position"=w654:sgl[])  [unwired: 2 in, 1 out]
          n199 = Equal To 0?(x=w635) -> (x = 0?=w634:bool)
          n200 = call "TraverseControl_High.vi"("Mode"=w653, "Route Checking?"=w652, "Home"=w645, "Traverse Name"=w651, "Extra command String"=w636, "Work in Tunnel Coordinates"=w633, "Model       Roll      Pitch       Yaw (deg)"=w648, "Final iteration of 3D_Trav Loop"=w634, "Position input XYZ"=w654, "Last Part of Move?"=w641, "Speed Factor"=w650, "Backlash Compensation?"=w646) -> ("Position Output XYZ"=w655:sgl[], "Error String"=w649:string)  [unwired: 2 in]
          n201 = Empty String/Path?(string/path=w649) -> (empty?=w647:bool)
        }
        n202 = case shown="\"Work in Model Coordinates\"" w610 {
          tunnel: w628 -> [w672 w675]
          tunnel: [w672 w674] -> w627
          tunnel: w629 -> [_ w673]
          frame "Work in Tunnel Coordinates" {
          }
          frame "Work in Model Coordinates" {
            n203 = call "Coordinate_rotation.vi"("Roll-Pitch-Yaw"=w673, "Input Position"=w675, "Mode"=T5."To User Coordinates") -> ("Output Position"=w674:sgl[])  [unwired: 2 in, 1 out]
          }
        }
      }
      frame "Update Position Globals" {
        n204 = case shown="\"Check VI only\"" w681 {
          tunnel: w680 -> [w691 _]
          tunnel: w679 -> [w690 _]
          tunnel: w678 -> [w689 _]
          tunnel: w677 -> [w688 _]
          frame "Check VI only" {
            n205 = stacked-sequence {
              seq-local: [w692 _] -> [_ w704]
              tunnel: w691 -> [_ w707]
              tunnel: w690 -> [w693 _]
              tunnel: w689 -> [w695 _]
              tunnel: w688 -> [w694 _]
              frame #0 {
                n206 = case shown="\"Work in Model Coordinates\"" w695 {
                  tunnel: w693 -> [w696 w699]
                  tunnel: [w696 w698] -> w692
                  tunnel: w694 -> [_ w697]
                  frame "Work in Tunnel Coordinates" {
                  }
                  frame "Work in Model Coordinates" {
                    n207 = call "Coordinate_rotation.vi"("Roll-Pitch-Yaw"=w697, "Input Position"=w699, "Mode"=T5."To Traverse Coordinates") -> ("Output Position"=w698:sgl[])  [unwired: 2 in, 1 out]
                  }
                }
              }
              frame #1 {
                n208 = global read "Trav_pos_global.vi" "Route checking Chs"() -> (w706:string[])
                n209 = global read "Trav_pos_global.vi" "ADAM Positions Ch names"() -> (w705:string[])
                n210 = for {
                  tunnel: w707 -> [w718]
                  tunnel: w706 -> [w717]
                  tunnel: w705 -> [w714]
                  tunnel: w704 -> [w713] mode=indexing
                  tunnel: [w712] -> w701 mode=indexing if=w708
                  tunnel: [w711] -> w702 mode=indexing if=w708
                  i -> [w720]
                  n211 = Format Into String(format string="%d", initial string=w718, w720) -> (resulting string=w716:string)  [unwired: 1 in, 1 out]
                  n212 = Search 1D Array(1D array=w717, element=w716) -> (index of element=w715:i32)  [unwired: 1 in]
                  n213 = Index Array(array=w714, index=w715) -> (element=w711:string)
                  n214 = Empty String/Path?(string/path=w711) -> (empty?=w709:bool)
                  n215 = Not(x=w709) -> (.not. x?=w708:bool)
                  n216 = Number To Fractional String(number=w713, precision (6)=i16 4) -> (F-format string=w712:string)  [unwired: 2 in]
                }
                n217 = call "Read_Write_Local_table_Quick.vi"("Mode"=Quick_local_ADAM_Table."Write Global", "String Values In"=w701, "Ch names In"=w702) -> ()  [unwired: 3 out]
              }
            }
          }
          frame "Run VI" {
          }
        }
        n218 = global write "Trav_pos_global.vi" "Traverse position"(w679) -> ()
        n219 = global write "Trav_pos_global.vi" "Live Position"(w679) -> ()
      }
      frame "Tidy up" {
        w721 = User_Specific_mode."Run VI" ("Simulate/Run")
        n220 = case shown="\"Move traverse\"" w726 {
          tunnel: w732 -> [w746 w813]
          tunnel: w731 -> [w747 w812]
          tunnel: w727 -> [w745 _]
          tunnel: [w744 w812] -> w730
          tunnel: w725 -> [w740 _]
          tunnel: w724 -> [w743 _]
          tunnel: w723 -> [w739 _]
          tunnel: w722 -> [w742 _]
          tunnel: w721 -> [w741 _]
          frame "Move traverse" {
            n221 = Equal?(x=w739, y=w741) -> (x = y?=w738:bool)
            n222 = And(x=w742, y=w738) -> (x .and. y?=w737:bool)
            n223 = case shown="False" w737 {
              tunnel: w747 -> [w752 w789]
              tunnel: w746 -> [w751 w792]
              tunnel: w745 -> [w750 _]
              tunnel: [w749 w787] -> w744
              tunnel: w743 -> [_ w786]
              tunnel: w740 -> [_ w783]
              frame False {
                n224 = Empty String/Path?(string/path=w752) -> (empty?=w748:bool)
                n225 = case shown="True" w748 {
                  tunnel: w751 -> [_ w757]
                  tunnel: w750 -> [_ w756]
                  tunnel: w752 -> [w753 w755]
                  tunnel: [w753 w754] -> w749
                  frame False {
                  }
                  frame True {
                    n226 = for {
                      tunnel: w757 -> [w760] mode=indexing
                      tunnel: w756 -> [w761] mode=indexing
                      shift-right: [w758] -> w754
                      shift-left: w755 -> [w759]
                      i -> [w764]
                      w766 = 10.0  # ±
                      n227 = case shown="0, Default" w764 {
                        tunnel: ["X" "Y" "Z"] -> w762
                        frame 0, Default {
                        }
                        frame 1 {
                        }
                        frame 2 {
                        }
                      }
                      n228 = call "In_Range_check.vi"("±"=w766, "Mode"=In_Range."±", "Value"=w761, "Setpoint"=w760) -> ("In Range"=w763:bool)  [unwired: 1 in, 2 out]
                      n229 = case shown="False" w763 {
                        tunnel: w762 -> [w773 _]
                        tunnel: w761 -> [w772 _]
                        tunnel: w760 -> [w771 _]
                        tunnel: w759 -> [w768 w774]
                        tunnel: [w769 w774] -> w758
                        frame False {
                          n230 = Format Into String(format string="For %s Axis Dem Pos = %.1f Achieved Pos = %.1f mm" ("Format String"), w773, w772, w771) -> (resulting string=w767:string)  [unwired: 2 in, 1 out]
                          n231 = Concatenate Strings(w768, w767) -> (w769:string)
                        }
                        frame True {
                        }
                      }
                    }
                  }
                }
              }
              frame True {
                n232 = local read "Position"() -> (w778:sgl[])
                n233 = case shown="\"Home  -X\"" w783 {
                  tunnel: [0 ("index") 0 ("index") 0 ("index") 1 ("index") 1 ("index") 2 ("index") 2 ("index")] -> w782
                  tunnel: ["-X" "+X" "-X" "+Y" "-Y" "+Z" "-Z"] -> w781
                  frame "Don't Home" {
                  }
                  frame "Home  +X" {
                  }
                  frame "Home  -X" {
                  }
                  frame "Home  +Y" {
                  }
                  frame "Home  -Y" {
                  }
                  frame "Home  +Z" {
                  }
                  frame "Home  -Z" {
                  }
                }
                n234 = Index Array(array=w792, index=w782) -> (element=w780:sgl)
                n235 = Index Array(array=w778, index=w782) -> (element=w779:sgl)
                n236 = Subtract(x=w780, y=w779) -> (x-y=w785:sgl)
                n237 = Multiply(x=0.995, y=w786) -> (x*y=w790:dbl)
                n238 = Absolute Value(x=w785) -> (abs(x)=w784:sgl)
                n239 = Less?(x=w784, y=w790) -> (x < y?=w788:bool)
                n240 = case shown="False" w788 {
                  tunnel: w789 -> [w810 w811]
                  tunnel: [w809 w811] -> w787
                  tunnel: w781 -> [w807 _]
                  frame False {
                    n241 = Concatenate Strings(w810, w807, " home has not been found.") -> (w809:string)
                  }
                  frame True {
                  }
                }
              }
            }
          }
          frame "Read traverse position", Default {
            n242 = local write "Position"(w813) -> ()
          }
        }
        n243 = local write "Currently on Point"(-1 ("Row Number")) -> ()
        n244 = local write "Simulate/Run"(w721) -> ()
      }
      frame "End" {
        n245 = case shown="Default" w814 {
          frame "Move traverse" {
          }
          frame Default {
            n246 = local write "Mode"(Trav_mode."Move traverse" ("Mode")) -> ()
            n247 = local write "Position Offset"(sgl[] [0.0, 0.0, 0.0] ("Position Offset")) -> ()
          }
        }
        n248 = case shown="\"Run VI\"" w821 {
          tunnel: w820 -> [_ w841]
          tunnel: w819 -> [_ w838]
          tunnel: w818 -> [_ w837]
          tunnel: w817 -> [_ w836]
          tunnel: w815 -> [w831 _]
          frame "Check VI only" {
            n249 = global read "Route_mapping_global.vi" "Display Mode"() -> (w833:T7)
            n250 = Equal?(x=w833, y=Route_Display_Mode."Display View Always" ("Display Mode")) -> (x = y?=w830:bool)
            n251 = And(x=w830, y=w831) -> (x .and. y?=w832:bool)
            n252 = case shown="True" w832 {
              frame False {
              }
              frame True {
                n253 = Wait (ms)(milliseconds to wait=u32 1500) -> ()  [unwired: 1 out]
              }
            }
          }
          frame "Run VI" {
            n254 = case shown="\"Work in Model Coordinates\"" w841 {
              tunnel: w838 -> [w842 w845]
              tunnel: [w842 w844] -> w839
              tunnel: w837 -> [_ w843]
              frame "Work in Tunnel Coordinates" {
              }
              frame "Work in Model Coordinates" {
                n255 = call "Coordinate_rotation.vi"("Roll-Pitch-Yaw"=w843, "Input Position"=w845, "Mode"=T5."To Traverse Coordinates") -> ("Output Position"=w844:sgl[])  [unwired: 2 in, 1 out]
              }
            }
            n256 = call "Read-Write_Check_Pos.vi"("Position input"=w839, "Mode"=enum16{"Read", "Write"}."Write", "Traverse Name"=w836) -> ()  [unwired: 1 out]
          }
        }
        n257 = local write "Route Checking?"(TRUE ("Route Checking?")) -> ()
        n258 = local write "Home"(Home."Don't Home" ("Home")) -> ()
      }
    }
  }
  "Trav Position achieved" <- w13
  "Error String" <- w17
